vi "TestTypeConversions.vi"() -> ()   [LabVIEW 2017]
panel:
  out "length":i32
  out "String":string
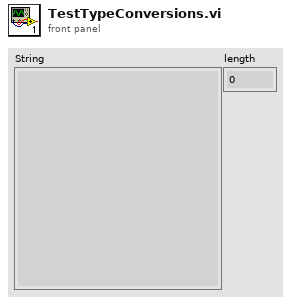
[diagram p1: front panel]
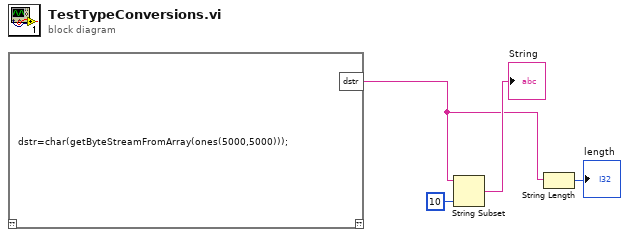
[diagram p0: block diagram]
diagram:
  n1 = script code="dstr=char(getByteStreamFromArray(ones(5000,5000)));"() -> ("dstr"=w2:string)  [unwired: 1 in, 1 out]
  n2 = String Subset(string=w2, length (rest)=10 ("length (rest)")) -> (substring=→"String":string)  [unwired: 1 in]
  n3 = String Length(string=w2) -> (length=→"length":i32)
